vi "Get ObjectType.vi"(8 "Error In":errorcluster, 11 "reference in":refnum<class "OD Entry.lvclass">) -> (0 "Error Out":errorcluster, 2 "ObjectType":T1 items=["NULL"=0, "DOMAIN"=2, "DEFTYPE"=5, "DEFSTRUCT"=6, "VAR"=7, "ARRAY"=8, "RECORD"=9], 3 "reference out":refnum<class "OD Entry.lvclass">)   [LabVIEW 2019, in "Electronic Datasheet.lvlib" / "OD Entry.lvclass"]
uses:
  OD Entry.lvclass
  Object Type/Object Type Base.lvclass
  Object Type.ctl
  Electronic Datasheet.lvlib
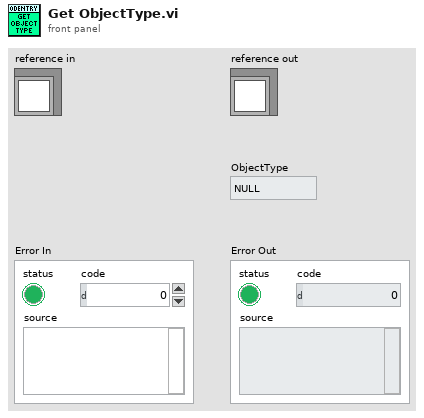
[diagram p1: front panel]
types:
  T1 = typedef "Electronic Datasheet.lvlib/Object Type.ctl" = u8
  T2 = typedef "Electronic Datasheet.lvlib/OD Entry.lvclass/ObjectAttributes.ctl" = cluster{"Index":u16, "ObjectType":refnum<class "Object Type Base.lvclass">, "Denotation":string, "Count":u8, "ObjExtend":u8, "Label":string, "Description":string, "PDO Mapping Type":T3, "Sub-Entries":map{u8, refnum<class "OD Sub-Entry.lvclass">}}
  T3 = typedef "Electronic Datasheet.lvlib/PDO Mapping Type.ctl" = enum16{"no", "optional", "RPDO", "TPDO", "UNKNOWN"}
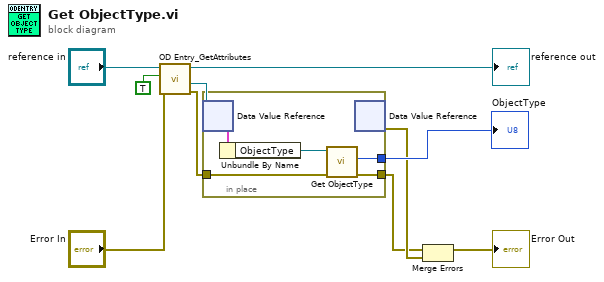
[diagram p0: block diagram]
diagram:
  n1 = call "OD Entry_GetAttributes.vi"("Error In"="Error In", "OnlyGetDvrReference(False)"=TRUE, "reference in"="reference in") -> ("Error Out"=w2:errorcluster, "DataRef"=w3:refnum<data-value>, "reference out"=→"reference out":refnum<class "OD Entry.lvclass">)  [unwired: 5 in, 1 out]
  n2 = in-place {
    in-place-border: w2 -> [w13]
    in-place-border: [w12] -> w1
    in-place-border: [w11] -> w6
    n3 = in-place-dvr #1(w3) -> (w14:T2)  [unwired: 1 out]
    n4 = Unbundle By Name(w14) -> ("ObjectType"=w15:refnum<class "Object Type Base.lvclass">)
    n5 = call-dynamic "Get ObjectType.vi"("error in"=w13, "Object Type in"=w15) -> ("error out"=w12:errorcluster, "ObjectType"=w11:T1)  [unwired: 6 in, 2 out]
    n6 = in-place-dvr #1() -> (w5:errorcluster)  [unwired: 1 in, 1 out]
  }
  "ObjectType" <- w6
  n7 = Merge Errors(w1, w5) -> (→"Error Out":errorcluster)
